vi "P4CMDSub Check for Installation.vi"(8 "error in (no error)":errorcluster) -> (0 "error out":errorcluster, 2 "path info":string, 5 "Perforce installed?":bool)   [LabVIEW 2017, in "NI_SCC_P4CMD.lvlib"]
uses:
  <vilib>/SourceControl/Providers/P4CMD/NI_SCC_P4CMD.lvlib
  <vilib>/SourceControl/support/SCCSup Message Strings GLBL.vi
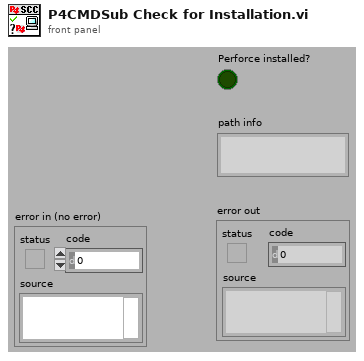
[diagram p1: front panel]
types:
  T1 = enum32{"invalid OS target", "Mac OS", "Windows 3.1", "Windows 95/NT", "Solaris 1", "Solaris 2", "HP-UX", "PowerMAX", "Linux", "Irix", "Rhapsody", "BeOS", "AIX", "OSF1", "VxWorks", "PharLap", "Carbon", "RTX", "Windows x64", "Linux x64", "Mac OS X x64"}
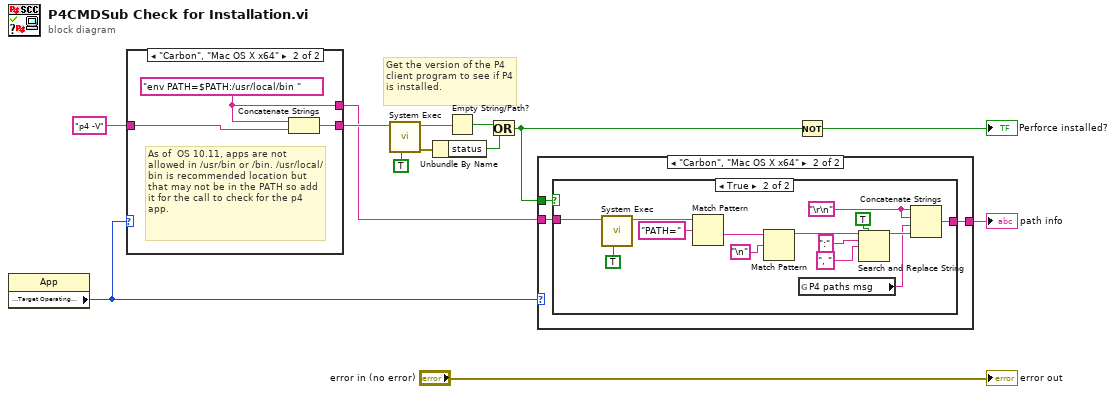
[diagram p0: block diagram]
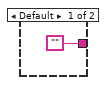
[diagram p3: hidden frame]
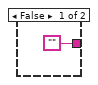
[diagram p4: hidden frame]
diagram:
  # "Get the version of the P4 client program to see if P4 is installed."
  n1 = property on="Property Node" class="App"() -> ("Application:Target Operating System"=w2:T1)  [unwired: 2 in, 2 out]
  n2 = case shown="\"Carbon\", \"Mac OS X x64\"" w2 {
    tunnel: "p4 -V" ("command line") -> [w14 w16]
    tunnel: [w14 w17] -> w3
    tunnel: [_ w15] -> w1
    frame Default {
    }
    frame "Carbon", "Mac OS X x64" {
      w15 = "env PATH=$PATH:/usr/local/bin " ("command line")
      # "As of  OS 10.11, apps are not allowed in /usr/bin or /bin. /usr/local/bin is recommended location but that may not be in the PATH so add it for the call to check for the p4 app."
      n3 = Concatenate Strings(w15, w16) -> (w17:string)
    }
  }
  n4 = call <vilib>:"System Exec.vi"("run minimized? (F)"=TRUE, "command line"=w3) -> ("error out"=w11:errorcluster, "standard output"=w12:string)  [unwired: 6 in, 2 out]
  n5 = Unbundle By Name(w11) -> ("status"=w13:bool)
  n6 = Empty String/Path?(string/path=w12) -> (empty?=w10:bool)
  n7 = Or(x=w10, y=w13) -> (x .or. y?=w5:bool)
  n8 = case shown="\"Carbon\", \"Mac OS X x64\"" w2 {
    tunnel: ["" ("Empty String Constant") w21] -> w7
    tunnel: w5 -> [_ w20]
    tunnel: w1 -> [_ w19]
    frame Default {
    }
    frame "Carbon", "Mac OS X x64" {
      n9 = case shown="True" w20 {
        tunnel: ["" ("Empty String Constant") w28] -> w21
        tunnel: w19 -> [_ w23]
        frame False {
        }
        frame True {
          w26 = "\r\n" ("End of Line Constant")
          n10 = call <vilib>:"System Exec.vi"("run minimized? (F)"=TRUE, "command line"=w23) -> ("standard output"=w35:string)  [unwired: 6 in, 3 out]
          n11 = Match Pattern(string=w35, regular expression="PATH=") -> (after substring=w33:string)  [unwired: 1 in, 3 out]
          n12 = Match Pattern(string=w33, regular expression="\n" ("Line Feed Constant")) -> (before substring=w32:string)  [unwired: 1 in, 3 out]
          n13 = global read "SCCSup Message Strings GLBL.vi" "P4 paths msg"() -> (w24:string)
          n14 = Search and Replace String(replace all?=TRUE ("replace all? (F)"), input string=w32, search string=":", replace string=", " ("replace string (\"\")")) -> (result string=w29:string)  [unwired: 4 in, 3 out]
          n15 = Concatenate Strings(w26, w26, w24, w29) -> (w28:string)
        }
      }
    }
  }
  "path info" <- w7
  n16 = Not(x=w5) -> (.not. x?=→"Perforce installed?":bool)
  "error out" <- "error in (no error)"
